vi "Compare IDs.vi"(10 "New IDs":set{i32}(c389), 11 "Current IDs":set{i32}(c389)) -> (1 "Result":T1(ring), 2 "Removed IDs":i32[](array[numeric]), 3 "Added IDs":i32[](array[numeric]))   [LabVIEW 2021, in "Seq Edit Quick Drop.lvlib"]
uses:
  Seq Edit Quick Drop.lvlib
  1e67f69e-a106-45ae-a325-7203d080973c.vi
  67f33a7c-9d8a-4da2-8438-0c57403dbbc6.vi
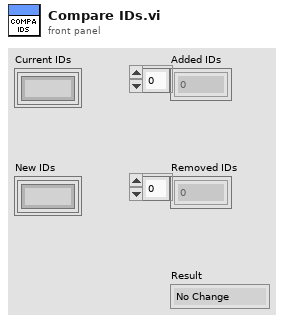
[diagram p1: front panel]
types:
  T1 = enum16{"No Change", "Added", "Removed", "Added and Removed"}
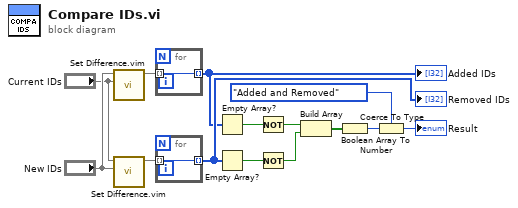
[diagram p0: block diagram]
diagram:
  n1 = call "Set Difference.vim"("set 2"="Current IDs", "set 1"="New IDs") -> ("difference"=w4:set{i32})  [unwired: 9 in]
  n2 = call "Set Difference.vim"("set 2"="New IDs", "set 1"="Current IDs") -> ("difference"=w14:set{i32})  [unwired: 9 in]
  n3 = for {
    tunnel: [w15] -> w3 mode=indexing
    tunnel: w4 -> [w15] mode=indexing
  }
  "Added IDs" <- w3
  n4 = for {
    tunnel: [w16] -> w13 mode=indexing
    tunnel: w14 -> [w16] mode=indexing
  }
  "Removed IDs" <- w13
  n5 = Empty Array?(array=w3) -> (empty?=w12:bool)
  n6 = Empty Array?(array=w13) -> (empty?=w11:bool)
  n7 = Not(x=w12) -> (.not. x?=w5:bool)
  n8 = Not(x=w11) -> (.not. x?=w6:bool)
  n9 = Build Array(w5, w6) -> (w10:bool[])
  n10 = Boolean Array To Number(Boolean array=w10) -> (number=w9:u32)
  n11 = Coerce To Type(0:w9, 1:T1."Added and Removed") -> (2:→"Result":T1)
